vi "Hardware In - NI 9751-4 (DI Driver).vi"(11 "FPGA Ref":T1) -> ()   [LabVIEW 2015, in "ECS-RT.lvlib"]
uses:
  ECS-RT.lvlib
  Typedefs/FPGA Refs/Generic FPGA Ref.ctl
  <vilib>/Utility/error.llb/Error Cluster From Error Code.vi
  <vilib>/rvi/errors/niLvFpgaAdjustHostInterfaceError.vi
  <vilib>/Powertrain Controls/Device Drivers/Tools/Real-Time/Interp1DTableRT.vi
  <vilib>/rvi/interface/nirviReadWriteControl/nirviReadWriteControl.xnode
  <vilib>/rvi/interface/Simulation/niFpgaSimulationCallBeginRW.vi
  NiFpgaLv.dll
  ECS-Shared.lvlib
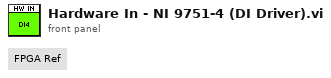
[diagram p1: front panel]
types:
  T1 = typedef "ECS-Shared.lvlib/Generic FPGA Ref.ctl" = refnum<k20>
  T2 = cluster{"ModulePresent":bool, "LVSense":u8, "HVSense":u8, "HVSense2":u8, "TempSense":i8, "Fault1":u8, "Fault2":u8, "OLIntegrator":u32, "HardwareRev":u8, "FirmwareRev":u8}
  T3 = cluster{"FI1OpenCircuit":bool, "FI2OpenCircuit":bool, "FI3OpenCircuit":bool}
  T4 = cluster{"PSCharge":bool, "PSOverLoad":bool, "ShortCircuit":bool, "ModuleTemperature":bool, "HighVoltageDriver":bool, "LowVoltageDriver":bool, "HighVoltageLimit":bool}
  T5 = cluster{"ModulePresent":bool, "Module Temperature (C)":sgl, "Internal High Voltage (V)":sgl, "External High Voltage (V)":sgl, "Battery Voltage (V)":sgl, "Hardware Rev":string, "Firmware Rev":u8}
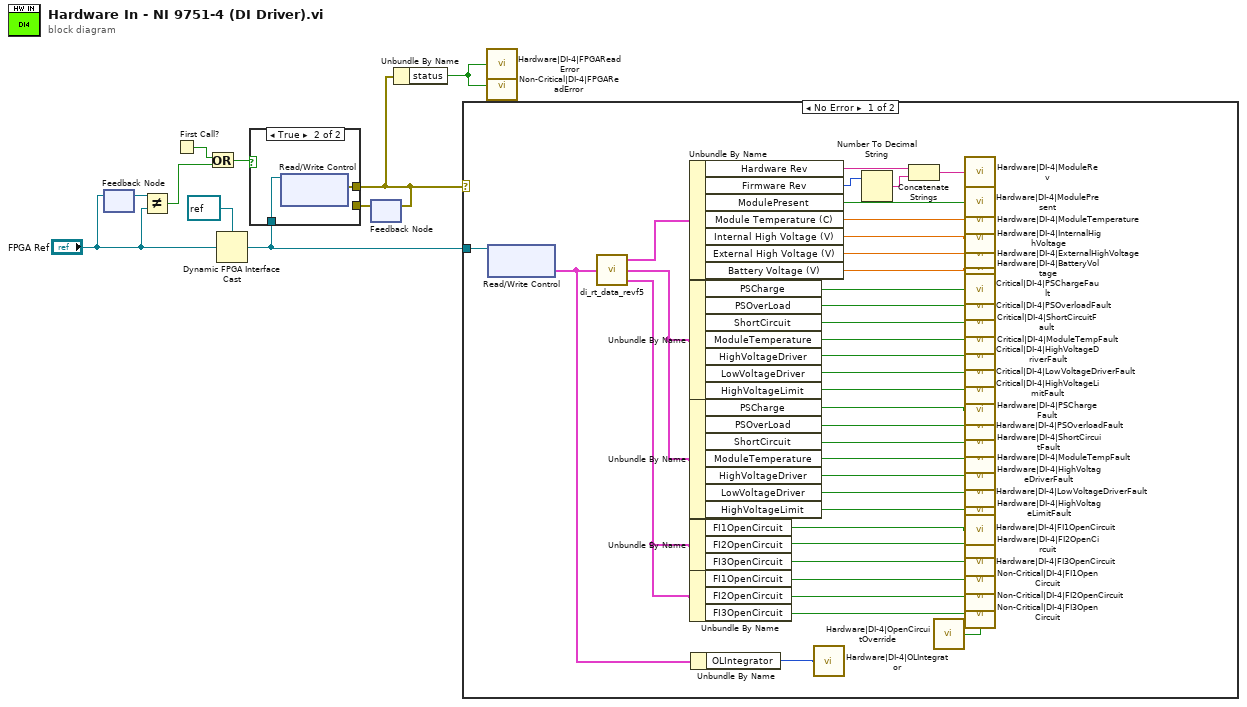
[diagram p0: block diagram]
diagram:
  n1 = feedback #1() -> (w9:T1)  [unwired: 1 in]
  n2 = feedback-in #1("FPGA Ref") -> ()
  n3 = Not Equal?(x=w9, y="FPGA Ref") -> (x != y?=w10:bool)
  n4 = First Call?() -> (First Call?: T/F=w8:bool)
  n5 = Or(x=w8, y=w10) -> (x .or. y?=w7:bool)
  n6 = Dynamic FPGA Interface Cast(Session In=refnum<k20> refnum ("FPGA VI Reference Out"), Type="FPGA Ref") -> (Session Out=w3:refnum<k20>)
  n7 = feedback #2() -> (w6:errorcluster)  [unwired: 1 in]
  n8 = case shown="True" w7 {
    tunnel: [w11 w13] -> w2
    tunnel: w6 -> [w11 _]
    tunnel: w3 -> [_ w12]
    frame False {
    }
    frame True {
      n9 = xnode "Read/Write Control"("FPGA VI Reference In"=w12) -> ("error out"=w13:errorcluster)  [unwired: 1 in, 2 out]
    }
  }
  n10 = feedback-in #2(w2) -> ()
  n11 = Unbundle By Name(w2) -> ("status"=w1:bool)
  n12 = case shown="No Error" w2 {
    tunnel: w3 -> [w14 _]
    frame No Error {
      n13 = xnode "Read/Write Control"("FPGA VI Reference In"=w14) -> ("DI-4.Data"=w15:T2)  [unwired: 1 in, 2 out]
      n14 = call <vilib>:"di_rt_data_revf5.vi"("DIDataFromFPGA"=w15) -> ("Non Critical Faults"=w45:T3, "Critical Faults"=w44:T4, "DIData"=w43:T5)  [unwired: 2 in]
      n15 = Unbundle By Name(w43) -> ("Hardware Rev"=w48:string, "Firmware Rev"=w49:u8, "ModulePresent"=w16:bool, "Module Temperature (C)"=w17:sgl, "Internal High Voltage (V)"=w18:sgl, "External High Voltage (V)"=w19:sgl, "Battery Voltage (V)"=w20:sgl)
      n16 = Unbundle By Name(w44) -> ("PSCharge"=w21:bool, "PSOverLoad"=w22:bool, "ShortCircuit"=w23:bool, "ModuleTemperature"=w24:bool, "HighVoltageDriver"=w25:bool, "LowVoltageDriver"=w26:bool, "HighVoltageLimit"=w27:bool)
      n17 = Unbundle By Name(w44) -> ("PSCharge"=w28:bool, "PSOverLoad"=w29:bool, "ShortCircuit"=w30:bool, "ModuleTemperature"=w31:bool, "HighVoltageDriver"=w32:bool, "LowVoltageDriver"=w33:bool, "HighVoltageLimit"=w34:bool)
      n18 = Unbundle By Name(w45) -> ("FI1OpenCircuit"=w35:bool, "FI2OpenCircuit"=w36:bool, "FI3OpenCircuit"=w37:bool)
      n19 = Unbundle By Name(w45) -> ("FI1OpenCircuit"=w38:bool, "FI2OpenCircuit"=w39:bool, "FI3OpenCircuit"=w40:bool)
      n20 = Unbundle By Name(w15) -> ("OLIntegrator"=w42:u32)
      n21 = call "Hardware|DI-4|OLIntegrator"("Value"=w42) -> ()
      n22 = Number To Decimal String(number=w49) -> (decimal integer string=w46:string)  [unwired: 1 in]
      n23 = Concatenate Strings(w48, w46) -> (w47:string)
      n24 = call "Hardware|DI-4|OpenCircuitOverride"() -> ("Value"=w41:bool)
      n25 = call "Hardware|DI-4|ModuleRev"("Value"=w47) -> ()
      n26 = call "Hardware|DI-4|ModulePresent"("Value"=w16) -> ()
      n27 = call "Hardware|DI-4|ModuleTemperature"("Value"=w17) -> ()
      n28 = call "Hardware|DI-4|InternalHighVoltage"("Value"=w18) -> ()
      n29 = call "Hardware|DI-4|ExternalHighVoltage"("Value"=w19) -> ()
      n30 = call "Hardware|DI-4|BatteryVoltage"("Value"=w20) -> ()
      n31 = call "Critical|DI-4|PSChargeFault"("Fault"=w21) -> ()  [unwired: 2 in]
      n32 = call "Critical|DI-4|PSOverloadFault"("Fault"=w22) -> ()  [unwired: 2 in]
      n33 = call "Critical|DI-4|ShortCircuitFault"("Fault"=w23) -> ()  [unwired: 2 in]
      n34 = call "Critical|DI-4|ModuleTempFault"("Fault"=w24) -> ()  [unwired: 2 in]
      n35 = call "Critical|DI-4|HighVoltageDriverFault"("Fault"=w25) -> ()  [unwired: 2 in]
      n36 = call "Critical|DI-4|LowVoltageDriverFault"("Fault"=w26) -> ()  [unwired: 2 in]
      n37 = call "Critical|DI-4|HighVoltageLimitFault"("Fault"=w27) -> ()  [unwired: 2 in]
      n38 = call "Hardware|DI-4|PSChargeFault"("Value"=w28) -> ()
      n39 = call "Hardware|DI-4|PSOverloadFault"("Value"=w29) -> ()
      n40 = call "Hardware|DI-4|ShortCircuitFault"("Value"=w30) -> ()
      n41 = call "Hardware|DI-4|ModuleTempFault"("Value"=w31) -> ()
      n42 = call "Hardware|DI-4|HighVoltageDriverFault"("Value"=w32) -> ()
      n43 = call "Hardware|DI-4|LowVoltageDriverFault"("Value"=w33) -> ()
      n44 = call "Hardware|DI-4|HighVoltageLimitFault"("Value"=w34) -> ()
      n45 = call "Hardware|DI-4|FI1OpenCircuit"("Value"=w35) -> ()
      n46 = call "Hardware|DI-4|FI2OpenCircuit"("Value"=w36) -> ()
      n47 = call "Hardware|DI-4|FI3OpenCircuit"("Value"=w37) -> ()
      n48 = call "Non-Critical|DI-4|FI1OpenCircuit"("Fault"=w38, "Override (F)"=w41) -> ()  [unwired: 1 in]
      n49 = call "Non-Critical|DI-4|FI2OpenCircuit"("Fault"=w39, "Override (F)"=w41) -> ()  [unwired: 1 in]
      n50 = call "Non-Critical|DI-4|FI3OpenCircuit"("Fault"=w40, "Override (F)"=w41) -> ()  [unwired: 1 in]
    }
    frame Error {
    }
  }
  n51 = call "Hardware|DI-4|FPGAReadError"("Value"=w1) -> ()
  n52 = call "Non-Critical|DI-4|FPGAReadError"("Fault"=w1) -> ()  [unwired: 2 in]
